vi "Start Timer.vi"(8 "error in (no error)":errorcluster, 10 "Duration":dbl, 11 "Motions in":refnum<class "Motions.lvclass">) -> (0 "error out":errorcluster, 3 "Motions out":refnum<class "Motions.lvclass">)   [LabVIEW 2016, in "Hardware.lvlib" / "Motions.lvlib" / "Motions.lvclass"]
uses:
  <userlib>/Common Components/Hardware/Abstract System/Motions/Motions/Motions.lvclass
  <userlib>/Common Components/Hardware/Abstract System/Motions/Motions/Motions.lvclass/Motions.ctl
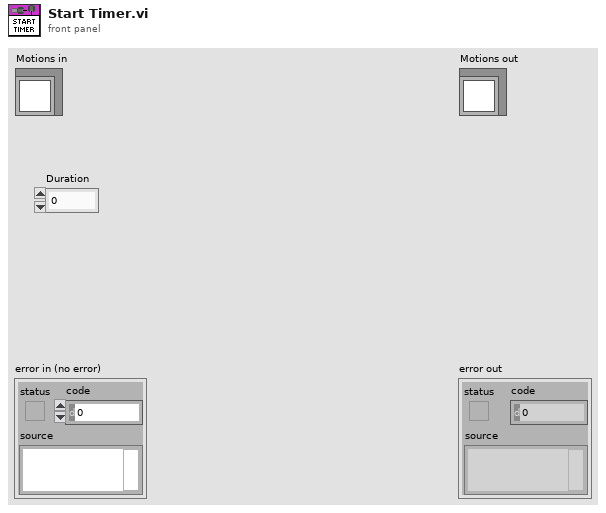
[diagram p1: front panel]
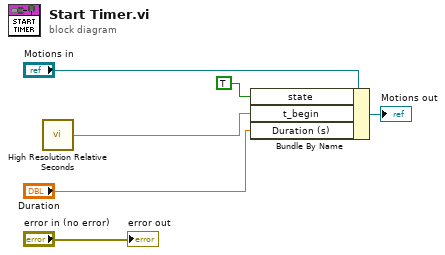
[diagram p0: block diagram]
diagram:
  n1 = call <vilib>:"High Resolution Relative Seconds.vi"() -> ("relative seconds"=w1:dbl)
  n2 = Bundle By Name(cluster="Motions in", "state"=TRUE ("Timer.state"), "t_begin"=w1, "Duration (s)"="Duration") -> (→"Motions out":refnum<class "Motions.lvclass">)
  "error out" <- "error in (no error)"
